vi "CLOSE.vi"(8 "error in (no error)":errorcluster, 11 "SERIAL DEVICE in":refnum<class "SERIAL DEVICE.lvclass">) -> (0 "error out":errorcluster, 3 "SERIAL DEVICE out":refnum<class "SERIAL DEVICE.lvclass">)   [LabVIEW 2019, in "SERIAL DEVICE.lvclass"]
uses:
  SERIAL DEVICE.lvclass
  SERIAL DEVICE.lvclass/SERIAL DEVICE.ctl
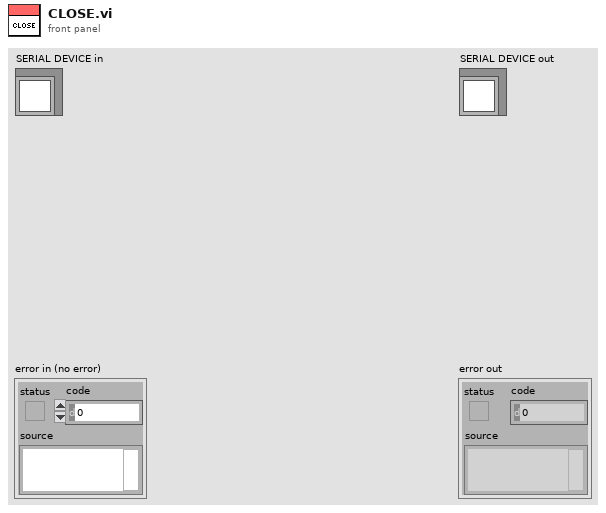
[diagram p1: front panel]
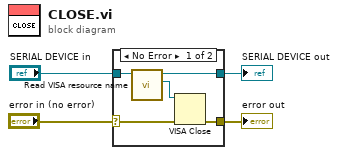
[diagram p0: block diagram]
diagram:
  n1 = case shown="No Error" "error in (no error)" {
    selector: "error in (no error)" -> [w6 w11]
    tunnel: [w5 w11] -> w3
    tunnel: [w8 w10] -> w1
    tunnel: "SERIAL DEVICE in" -> [w9 w10]
    frame No Error {
      n2 = call "Read VISA resource name.vi"("SERIAL DEVICE in"=w9) -> ("VISA resource name"=w7:refnum<visa-resource-name>, "SERIAL DEVICE out"=w8:refnum<class "SERIAL DEVICE.lvclass">)  [unwired: 8 in, 1 out]
      n3 = VISA Close(VISA resource name=w7, error in (no error)=w6) -> (error out=w5:errorcluster)
    }
    frame Error {
    }
  }
  "error out" <- w3
  "SERIAL DEVICE out" <- w1
